vi "Write Secure.vi"(8 "error in (no error)":errorcluster, 10 "Secure":bool, 11 "WebSocket Server Manager in":refnum<class "WebSocket Server Manager.lvclass">) -> (0 "error out":errorcluster, 3 "WebSocket Server Manager out":refnum<class "WebSocket Server Manager.lvclass">)   [LabVIEW 2021, in "WebSocket Actors.lvlib" / "WebSocket Server Manager.lvclass"]
uses:
  WebSocket Server Manager.lvclass
  WebSocket Server Manager.lvclass/WebSocket Server Manager.ctl
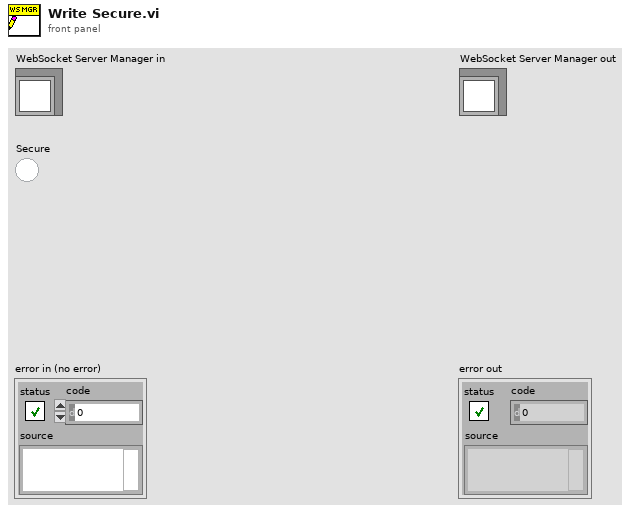
[diagram p1: front panel]
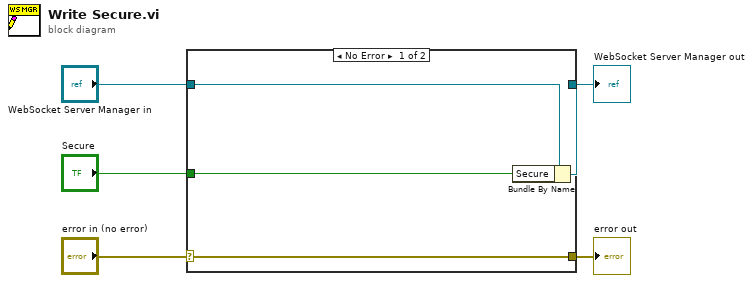
[diagram p0: block diagram]
diagram:
  n1 = case shown="No Error" "error in (no error)" {
    selector: "error in (no error)" -> [w9 w10]
    tunnel: [w9 w10] -> w4
    tunnel: [w7 w11] -> w2
    tunnel: "WebSocket Server Manager in" -> [w8 w11]
    tunnel: "Secure" -> [w6 _]
    frame No Error {
      n2 = Bundle By Name(cluster=w8, "Secure"=w6) -> (w7:refnum<class "WebSocket Server Manager.lvclass">)
    }
    frame Error {
    }
  }
  "error out" <- w4
  "WebSocket Server Manager out" <- w2
